vi "DecreaseFrame.vi"   [LabVIEW 2014]
uses:
  USBAnalyzerEllisysDll/Debug/USBAnalyzerEllisysDll.dll
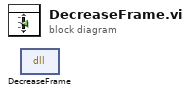
[diagram p0: block diagram]
diagram:
  n1 = dll-call lib="PTH2labs CUsersMichał\tDocumentsEllisysAnalyzerUSBAnalyzerEllisysDllDebugUSBAnalyzerEllisysDll.dll" fn="DecreaseFrame"() -> ()  [unwired: 4 in, 2 out]
